vi "Close.vi"(8 "error in (no error)":errorcluster, 11 "VISA TCP in":refnum<class "VISA TCP.lvclass">) -> (0 "error out":errorcluster)   [LabVIEW 2013, in "Sockets.lvlib" / "VISA TCP.lvclass"]
doc: "Closes the socket connection."
uses:
  VISA TCP.lvclass
  VISA TCP.lvclass/VISA TCP.ctl
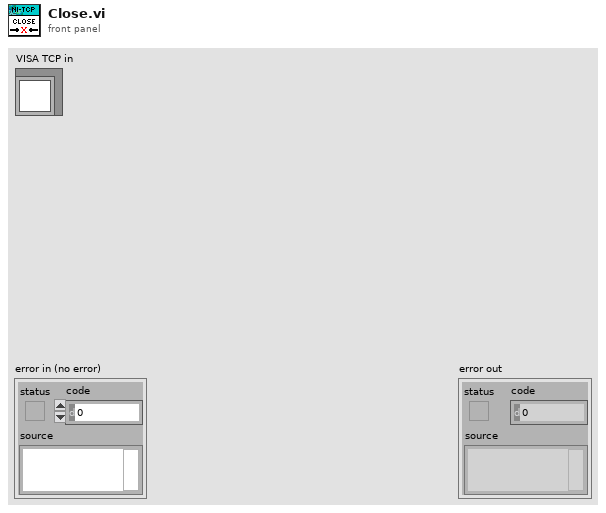
[diagram p1: front panel]
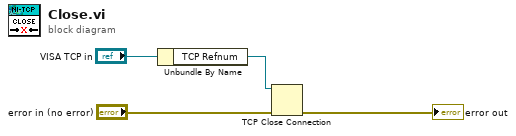
[diagram p0: block diagram]
diagram:
  n1 = Unbundle By Name("VISA TCP in") -> ("TCP Refnum"=w1:refnum<k5>)
  n2 = TCP Close Connection(connection ID=w1, error in (no error)="error in (no error)") -> (error out=→"error out":errorcluster)  [unwired: 1 in, 1 out]
